vi "ISEG_HVChannel.set Refresh Status.vi"(0 "i ref in":refnum<vi>, 5 "Refresh rate":i32, 7 "Force":bool, 11 "error in (no error)":errorcluster) -> (4 "i ref out":refnum<vi>, 15 "error out":errorcluster)   [LabVIEW 2014, in "ISEG_HVChannel.lvlib"]
doc: "this vi set the default values for force_status and refresh rate."
uses:
  ISEG_HVChannel.lvlib
  CS_Core/CSSystem/CoreLib/CoreLib.string 2 byte array.vi
  CS_Core/CSSystem/CoreLib/CoreLib.short 2 byte array.vi
  CS_Core/CSSystem/CoreLib/CoreLib.double 2 byte array.vi
  CS_Core/BaseProcess/BaseProcess.lvlib
  CS_Core/CSSystem/CoreLib/CoreLib.lvlib
  CSlibraries-extern/DimLVEvent/LVDimInterface/LVDimInterface.lvlib
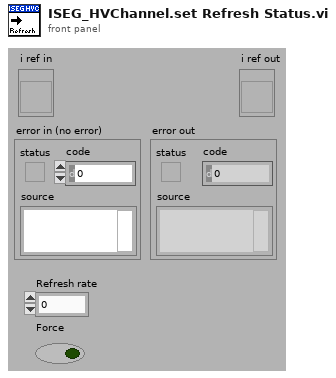
[diagram p1: front panel]
types:
  T1 = typedef "BaseProcess.lvlib/BaseProcess.i attribute.ctl" = cluster{"EventStatus":string, "EventError":i32, "PresetEvtWatchD":i32, "PresetPdcWatchD":i32, "EventTimeout":i32, "PeriodicInterval":i32, "Interface":string[], "Address":string[], "Special":string[], "PeriodicError":i32, "PeriodicStatus":string, "SuperProc":string, "Descriptors":T2[], "CaseRef":refnum<vi>, "PdcRef":refnum<vi>, "Thread Ref":refnum<vi>, "eventErrorID":i32, "eventStatusID":i32, "periodicErrorID":i32, "periodicStatusID":i32, "pdcCtrID":i32}
  T2 = typedef "BaseProcess.lvlib/BaseProcess.descriptor definition.ctl" = cluster{"selector":string, "descriptor":T3}
  T3 = typedef "BaseProcess.lvlib/BaseProcess.descriptor string definition.ctl" = string
  T4 = typedef "CoreDefs.rawDataType.ctl" = i8[]
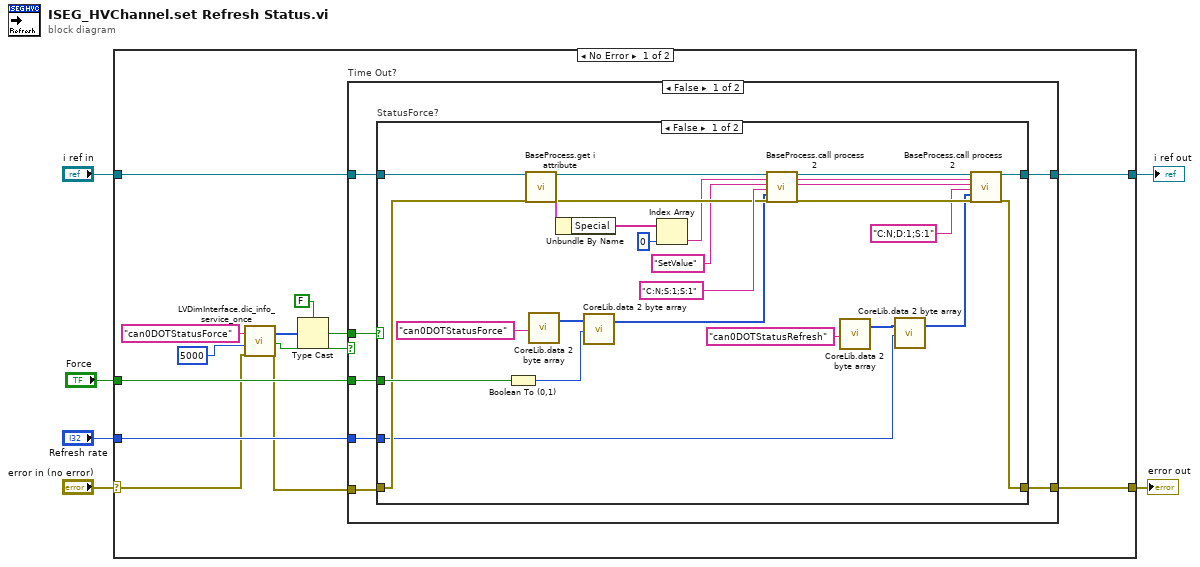
[diagram p0: block diagram]
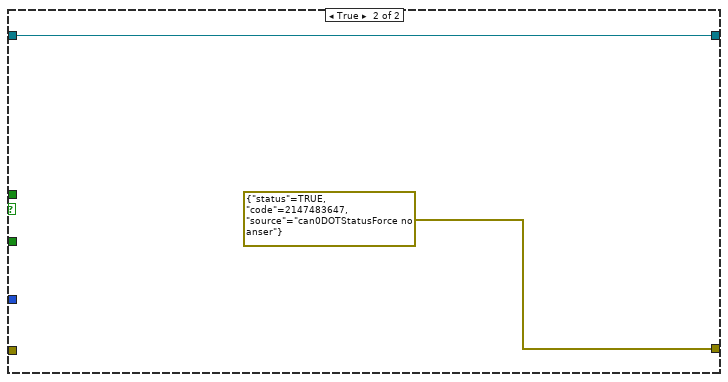
[diagram p3: hidden frame]
diagram:
  n1 = case shown="No Error" "error in (no error)" {
    selector: "error in (no error)" -> [w10 w55]
    tunnel: "i ref in" -> [w19 w56]
    tunnel: "Refresh rate" -> [w18 _]
    tunnel: "Force" -> [w15 _]
    tunnel: [w17 w56] -> w2
    tunnel: [w16 w55] -> w1
    frame No Error {
      n2 = call "LVDimInterface.dic_info_service_once.vi"("serviceName"="can0DOTStatusForce", "timeout [ms]"=u32 5000, "error in (no error)"=w10) -> ("data"=w12:i8[], "timed out?"=w7:bool, "error out"=w9:errorcluster)  [unwired: 13 in, 1 out]
      n3 = Type Cast(type=FALSE, x=w12) -> (*(type *) &x=w11:bool)
      n4 = case "Time Out?" shown="False" w7 {
        tunnel: w19 -> [w26 w53]
        tunnel: w18 -> [w25 _]
        tunnel: [w24 w53] -> w17
        tunnel: [w23 errorcluster {"status"=TRUE, "code"=2147483647, "source"="can0DOTStatusForce no anser"} ("error out")] -> w16
        tunnel: w15 -> [w22 _]
        tunnel: w11 -> [w21 _]
        tunnel: w9 -> [w20 _]
        frame False {
          n5 = case "StatusForce?" shown="False" w21 {
            tunnel: w26 -> [w50 w52]
            tunnel: w25 -> [w28 _]
            tunnel: [w42 w52] -> w24
            tunnel: [w40 w51] -> w23
            tunnel: w22 -> [w35 _]
            tunnel: w20 -> [w34 w51]
            frame False {
              w38 = "SetValue" ("Selector")
              n6 = Boolean To (0,1)(Boolean=w35) -> (0, 1=w32:i16)
              n7 = call "BaseProcess.get i attribute.vi"("i ref in"=w50, "error in (no error)"=w34) -> ("i ref out"=w45:refnum<vi>, "i attribute"=w47:T1, "error out"=w44:errorcluster)  [unwired: 15 in]
              n8 = call-poly "CoreLib.data 2 byte array.vi"("string"="can0DOTStatusForce") -> ("byteArray out"=w31:T4)  [unwired: 18 in]
              n9 = Unbundle By Name(w47) -> ("Special"=w49:string[])
              n10 = call-poly "CoreLib.data 2 byte array.vi"("byteArray"=w31, "i16"=w32) -> ("byteArray out"=w27:T4)  [unwired: 17 in]
              n11 = Index Array(array=w49, index=0) -> (element=w39:string)
              n12 = call "BaseProcess.call process 2.vi"("i ref in"=w45, "Object"=w39, "Selector"=w38, "Data Descriptor"="C:N;S:1;S:1", "Data"=w27, "error in (no error)"=w44) -> ("i ref out"=w43:refnum<vi>, "error out"=w41:errorcluster)  [unwired: 12 in]
              n13 = call-poly "CoreLib.data 2 byte array.vi"("string"="can0DOTStatusRefresh") -> ("byteArray out"=w30:T4)  [unwired: 18 in]
              n14 = call-poly "CoreLib.data 2 byte array.vi"("byteArray"=w30, "f64"=w28) -> ("byteArray out"=w29:T4)  [unwired: 17 in]
              n15 = call "BaseProcess.call process 2.vi"("i ref in"=w43, "Object"=w39, "Selector"=w38, "Data Descriptor"="C:N;D:1;S:1", "Data"=w29, "error in (no error)"=w41) -> ("i ref out"=w42:refnum<vi>, "error out"=w40:errorcluster)  [unwired: 12 in]
            }
            frame True {
            }
          }
        }
        frame True {
        }
      }
    }
    frame Error {
    }
  }
  "error out" <- w1
  "i ref out" <- w2
